vi "Test1.vi"() -> ()   [LabVIEW 2020]
uses:
  Postgres Connector/Cluster_Return_Of_The_Query.ctl
  Postgres Connector/Postgres Connector.lvclass
panel:
  out "Q Time":u32
  out "Query Return":T1[](array[typedef])
  in  "Query String":string="select pg_size_pretty(pg_database_size('postgres')) as size;\n"
  in  "Query":bool
  out "Hours":dbl
  out "Status":bool
  in  "Start Insert":bool
  out "Insert Time":u32(graph)
  in  "Count":i32=2000
  in  "Connect":bool
  in  "Connection Info":T2={"IP Address"="192.168.5.50", "Port"=5432, "Timeout"=2000, "User"="postgres", "Password"="28779867", "Database"="postgres"}
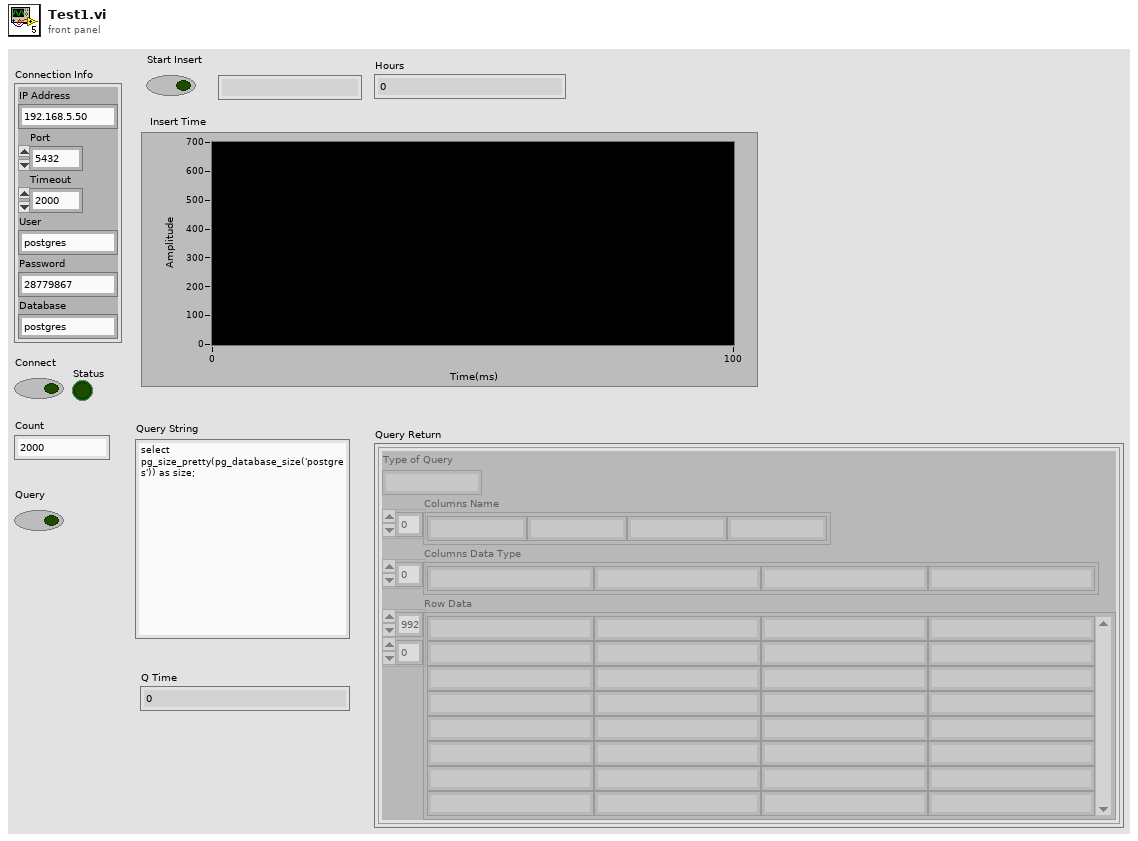
[diagram p1: front panel]
types:
  T1 = typedef "Postgres Connector.lvclass/Cluster_Return_Of_The_Query.ctl" = cluster{"Type of Query":string, "Columns Name":string[], "Columns Data Type":string[], "Row Data":string[][]}
  T2 = cluster{"IP Address":string, "Port":u16, "Timeout":i32, "User":string, "Password":string, "Database":string}
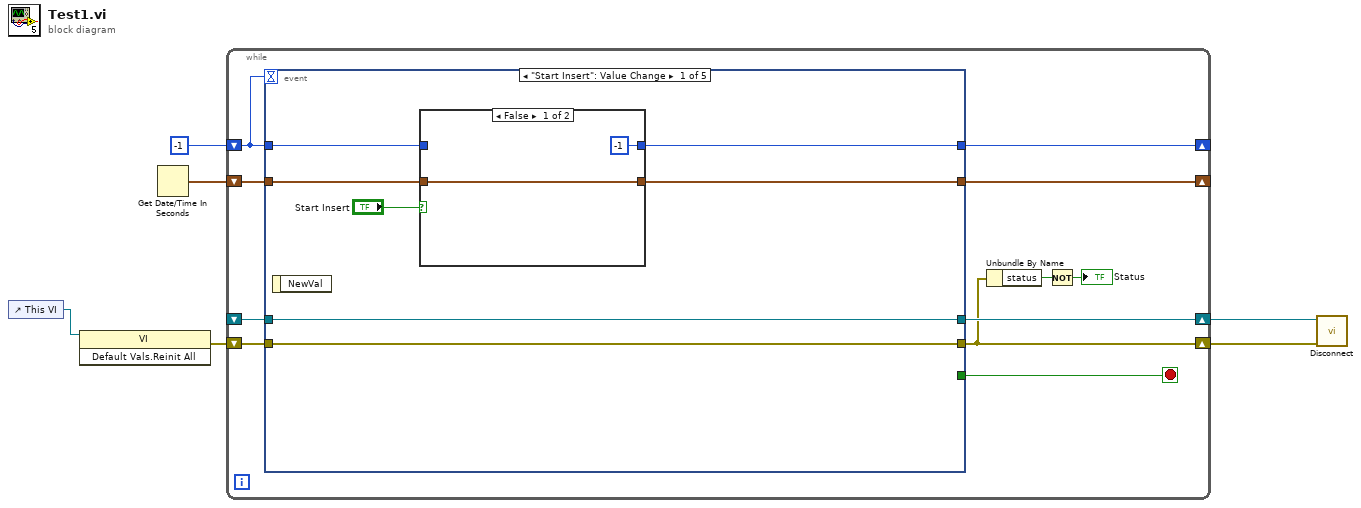
[diagram p0: block diagram]
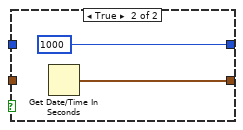
[diagram p2: hidden frame]
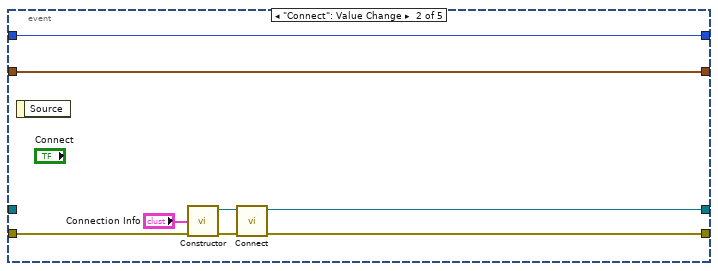
[diagram p3: hidden frame]
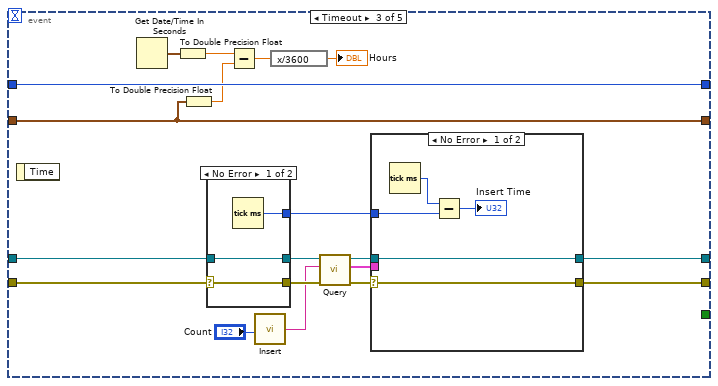
[diagram p4: hidden frame]
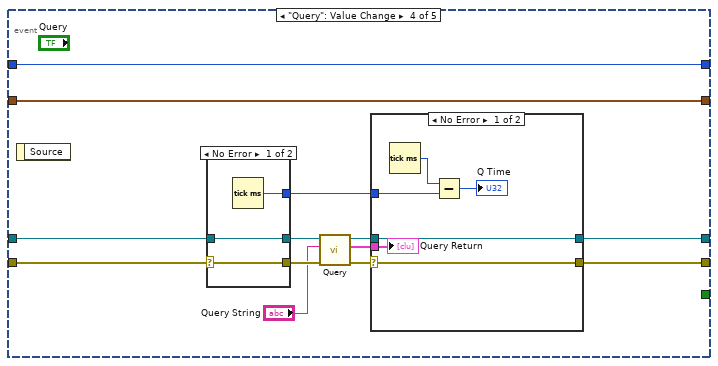
[diagram p7: hidden frame]
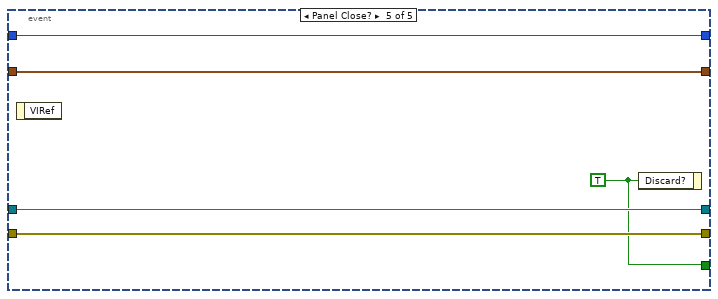
[diagram p10: hidden frame]
diagram:
  n1 = control-ref of="This VI"() -> (w1:refnum<vi>)
  n2 = invoke class="VI" method="Default Vals.Reinit All"(reference=w1) -> (error out=w2:errorcluster)  [unwired: 2 in, 2 out]
  n3 = Get Date/Time In Seconds() -> (seconds since 1Jan1904=w3:timestamp)
  n4 = while {
    shift-right: [w11] -> w6
    shift-left: w2 -> [w17]
    shift-right: [w16] -> w5
    shift-left: _ -> [w14]
    shift-right: [w12] -> _
    shift-left: -1 -> [w13]
    shift-right: [w7] -> _
    shift-left: w3 -> [w8]
    stop <- w15 stop-if-true
    n5 = event shown="[0] \"Start Insert\": Value Change" {
      selector: _ -> [_ _ _ _ _]
      dyn-events: _ -> [_ _ _ _ _]
      timeout: w13 -> [_ _ _ _ _]
      tunnel: w17 -> [w22 w33 w55 w80 w98]
      tunnel: w14 -> [w23 _ w53 w78 w97]
      tunnel: [w22 w32 w49 w74 w98] -> w11
      tunnel: [w23 w31 w48 w73 w97] -> w16
      tunnel: [_ _ _ _ w96] -> w15
      tunnel: w13 -> [w21 w30 w45 w70 w94]
      tunnel: [w20 w30 w45 w70 w94] -> w12
      tunnel: w8 -> [w18 w29 w41 w69 w95]
      tunnel: [w19 w29 w41 w69 w95] -> w7
      event "Start Insert": Value Change {
        n6 = event-data() -> ()  [unwired: 1 in, 1 out]
        n7 = case shown="False" "Start Insert" {
          tunnel: w21 -> [_ _]
          tunnel: [-1 1000] -> w20
          tunnel: [w25 w27] -> w19
          tunnel: w18 -> [w25 _]
          frame False {
          }
          frame True {
            n8 = Get Date/Time In Seconds() -> (seconds since 1Jan1904=w27:timestamp)
          }
        }
      }
      event "Connect": Value Change {
        n9 = event-data() -> ()  [unwired: 1 in, 1 out]
        n10 = call "Constructor.vi"("error in (no error)"=w33, "Connection Info"="Connection Info") -> ("error out"=w34:errorcluster, "Postgres Connector Out"=w35:refnum<class "Postgres Connector.lvclass">)  [unwired: 8 in]
        n11 = call "Connect.vi"("error in (no error)"=w34, "Postgres Connector In"=w35) -> ("error out"=w32:errorcluster, "Postgres Connector Out"=w31:refnum<class "Postgres Connector.lvclass">)  [unwired: 8 in]
      }
      event Timeout {
        n12 = event-data() -> ()  [unwired: 1 in, 1 out]
        n13 = Get Date/Time In Seconds() -> (seconds since 1Jan1904=w42:timestamp)
        n14 = To Double Precision Float(number=w42) -> (double precision float=w40:dbl)
        n15 = To Double Precision Float(number=w41) -> (double precision float=w39:dbl)
        n16 = case shown="No Error" w55 {
          selector: w55 -> [w65 w67]
          tunnel: [w65 w67] -> w54
          tunnel: w53 -> [w64 w66]
          tunnel: [w64 w66] -> w52
          tunnel: [w63 _] -> w47
          frame No Error {
            n17 = Tick Count (ms)() -> (millisecond timer value=w63:u32)
          }
          frame Error {
          }
        }
        n18 = Subtract(x=w40, y=w39) -> (x-y=w38:dbl)
        n19 = call "Insert.vi"("Count"="Count") -> ("Inser String"=w43:string)
        n20 = expression code="x/3600"(w38) -> (→"Hours":dbl)
        n21 = call "Query.vi"("error in (no error)"=w54, "Query"=w43, "Postgres Connector In"=w52) -> ("error out"=w51:errorcluster, "Query Return"=w46:T1[], "Postgres Connector Out"=w50:refnum<class "Postgres Connector.lvclass">)  [unwired: 6 in]
        n22 = case shown="No Error" w51 {
          selector: w51 -> [w60 w62]
          tunnel: [w60 w62] -> w49
          tunnel: w50 -> [w59 w61]
          tunnel: [w59 w61] -> w48
          tunnel: w47 -> [w58 _]
          tunnel: w46 -> [_ _]
          frame No Error {
            n23 = Tick Count (ms)() -> (millisecond timer value=w57:u32)
            n24 = Subtract(x=w57, y=w58) -> (x-y=→"Insert Time":u32)
          }
          frame Error {
          }
        }
      }
      event "Query": Value Change {
        n25 = event-data() -> ()  [unwired: 1 in, 1 out]
        n26 = case shown="No Error" w80 {
          selector: w80 -> [w91 w93]
          tunnel: [w91 w93] -> w79
          tunnel: w78 -> [w90 w92]
          tunnel: [w90 w92] -> w77
          tunnel: [w89 _] -> w72
          frame No Error {
            n27 = Tick Count (ms)() -> (millisecond timer value=w89:u32)
          }
          frame Error {
          }
        }
        n28 = call "Query.vi"("error in (no error)"=w79, "Query"="Query String", "Postgres Connector In"=w77) -> ("error out"=w76:errorcluster, "Query Return"=w71:T1[], "Postgres Connector Out"=w75:refnum<class "Postgres Connector.lvclass">)  [unwired: 6 in]
        n29 = case shown="No Error" w76 {
          selector: w76 -> [w86 w88]
          tunnel: [w86 w88] -> w74
          tunnel: w75 -> [w85 w87]
          tunnel: [w85 w87] -> w73
          tunnel: w72 -> [w84 _]
          tunnel: w71 -> [w82 _]
          frame No Error {
            n30 = Tick Count (ms)() -> (millisecond timer value=w83:u32)
            n31 = Subtract(x=w83, y=w84) -> (x-y=→"Q Time":u32)
            "Query Return" <- w82
          }
          frame Error {
          }
        }
      }
      event Panel Close? {
        w96 = TRUE ("Discard?")
        n32 = event-data() -> ()  [unwired: 1 in, 1 out]
        n33 = event-data("Discard?"=w96) -> ()  [unwired: 1 in, 1 out]
      }
    }
    n34 = Unbundle By Name(w11) -> ("status"=w10:bool)
    n35 = Not(x=w10) -> (.not. x?=→"Status":bool)
  }
  n36 = call "Disconnect.vi"("error in (no error)"=w6, "Postgres Connector In"=w5) -> ()  [unwired: 8 in, 2 out]
